vi "Convert taus and time.vi"   [LabVIEW 2012]
types:
  T1 = enum16{"open", "replace", "create", "open or create", "replace or create", "replace or create with confirmation"}
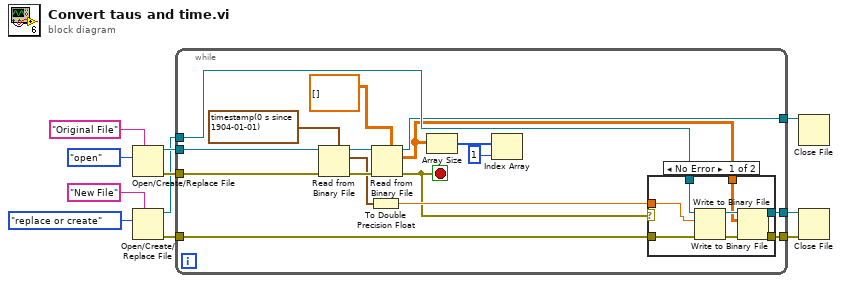
[diagram p0: block diagram]
diagram:
  n1 = Open/Create/Replace File(prompt="Original File", operation (0:open)=T1."open") -> (refnum out=w11:refnum<file>, error out=w10:errorcluster)  [unwired: 4 in, 1 out]
  n2 = Open/Create/Replace File(prompt="New File", operation (0:open)=T1."replace or create") -> (refnum out=w9:refnum<file>, error out=w8:errorcluster)  [unwired: 4 in, 1 out]
  n3 = while {
    tunnel: w11 -> [w28]
    tunnel: w10 -> [w27]
    tunnel: w9 -> [w22]
    tunnel: w8 -> [w21]
    tunnel: [w16] -> w7
    tunnel: [w15] -> w6
    tunnel: [w14] -> w5
    stop <- w12 stop-if-true
    n4 = Read from Binary File(5:timestamp(0 s since 1904-01-01), 8:w27, 11:w28) -> (0:w25:errorcluster, 2:w20:timestamp, 3:w26:refnum<file>)  [unwired: 3 in, 1 out]
    n5 = To Double Precision Float(number=w20) -> (double precision float=w13:dbl)
    n6 = Read from Binary File(5:dbl[][] [], 8:w25, 11:w26) -> (0:w12:errorcluster, 2:w19:dbl[][], 3:w14:refnum<file>)  [unwired: 3 in, 1 out]
    n7 = Array Size(array=w19) -> (size(s)=w18:i32[])
    n8 = Index Array(array=w18, index=1) -> ()  [unwired: 1 out]
    n9 = case shown="No Error" w12 {
      tunnel: w22 -> [w36 w38]
      tunnel: w21 -> [w35 w37]
      tunnel: w19 -> [w32 _]
      tunnel: [w31 w37] -> w16
      tunnel: [w30 w38] -> w15
      tunnel: w13 -> [w29 _]
      frame No Error {
        n10 = Write to Binary File(file (use dialog)=w36, data=w29, error in=w35) -> (refnum out=w34:refnum<file>, error out=w33:errorcluster)  [unwired: 3 in, 1 out]
        n11 = Write to Binary File(file (use dialog)=w34, data=w32, error in=w33) -> (refnum out=w30:refnum<file>, error out=w31:errorcluster)  [unwired: 3 in, 1 out]
      }
      frame Error {
      }
    }
  }
  n12 = Close File(refnum=w5) -> ()  [unwired: 1 in, 2 out]
  n13 = Close File(refnum=w6, error in=w7) -> ()  [unwired: 2 out]
